vi "Logger Set Viewer Run Mode.vi"(0 "Server Status":enum16{"Running", "Closed"}(ring), 11 "error in (no error)":errorcluster) -> (15 "error out":errorcluster)   [LabVIEW 2018]
uses:
  Logger Global.vi
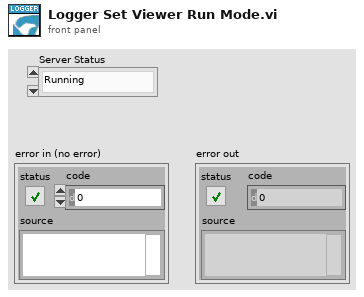
[diagram p1: front panel]
types:
  T1 = enum32{"Invalid", "Standard", "Closed", "Hidden", "Minimized", "Maximized"}
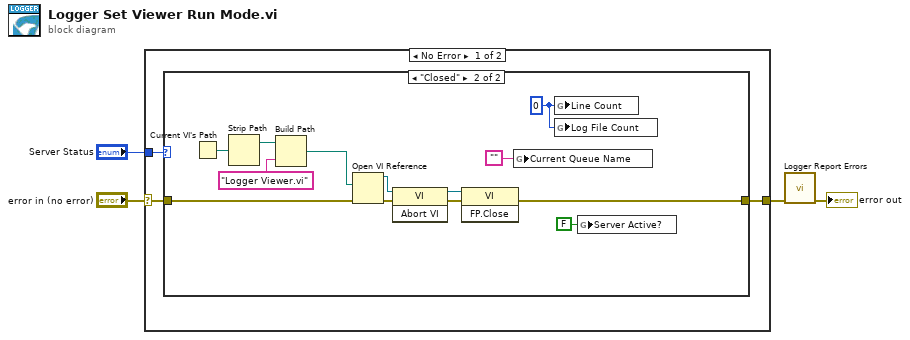
[diagram p0: block diagram]
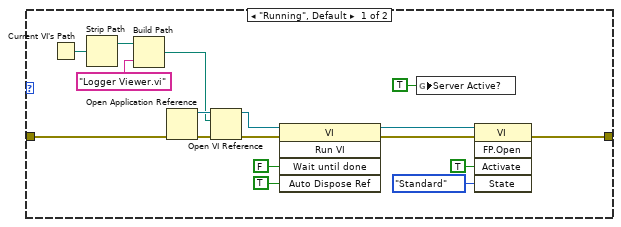
[diagram p2: hidden frame]
diagram:
  n1 = case shown="No Error" "error in (no error)" {
    selector: "error in (no error)" -> [w7 w38]
    tunnel: [w6 w38] -> w2
    tunnel: "Server Status" -> [w5 _]
    frame No Error {
      n2 = case shown="\"Closed\"" w5 {
        tunnel: w7 -> [w24 w35]
        tunnel: [w15 w34] -> w6
        frame "Running", Default {
          n3 = Current VI's Path() -> (path=w12:path)
          n4 = Strip Path(path=w12) -> (stripped path=w11:path)  [unwired: 1 out]
          n5 = Build Path(base path=w11, name or relative path="Logger Viewer.vi") -> (appended path=w9:path)
          n6 = Open Application Reference(8:w24) -> (0:w22:errorcluster, 3:w23:refnum<vi>)  [unwired: 3 in]
          n7 = Open VI Reference(application reference (local)=w23, vi path=w9, error in (no error)=w22) -> (vi reference=w20:refnum<vi>, error out=w21:errorcluster)  [unwired: 3 in]
          n8 = invoke class="VI" method="Run VI"(reference=w20, error in=w21, "Wait until done"=FALSE ("Wait Until Done"), "Auto Dispose Ref"=TRUE ("Auto Dispose Reference")) -> (reference out=w16:refnum<vi>, error out=w17:errorcluster)  [unwired: 1 in, 3 out]
          n9 = global write "Logger Global.vi" "Server Active?"(TRUE ("Server Active?")) -> ()
          n10 = invoke class="VI" method="FP.Open"(reference=w16, error in=w17, "Activate"=TRUE ("Activate?"), "State"=T1."Standard") -> (error out=w15:errorcluster)  [unwired: 1 in, 4 out]
        }
        frame "Closed" {
          w26 = u16 0 ("Line Count")
          n11 = Current VI's Path() -> (path=w31:path)
          n12 = Strip Path(path=w31) -> (stripped path=w30:path)  [unwired: 1 out]
          n13 = Build Path(base path=w30, name or relative path="Logger Viewer.vi") -> (appended path=w28:path)
          n14 = Open VI Reference(vi path=w28, error in (no error)=w35) -> (vi reference=w36:refnum<vi>, error out=w37:errorcluster)  [unwired: 4 in]
          n15 = invoke class="VI" method="Abort VI"(reference=w36, error in=w37) -> (reference out=w32:refnum<vi>, error out=w33:errorcluster)  [unwired: 1 in, 1 out]
          n16 = invoke class="VI" method="FP.Close"(reference=w32, error in=w33) -> (error out=w34:errorcluster)  [unwired: 1 in, 2 out]
          n17 = global write "Logger Global.vi" "Current Queue Name"("") -> ()
          n18 = global write "Logger Global.vi" "Line Count"(w26) -> ()
          n19 = global write "Logger Global.vi" "Log File Count"(w26) -> ()
          n20 = global write "Logger Global.vi" "Server Active?"(FALSE ("Server Status")) -> ()
        }
      }
    }
    frame Error {
    }
  }
  n21 = call "Logger Report Errors.vi"("error in (no error)"=w2) -> ("error out"=→"error out":errorcluster)  [unwired: 14 in]
